vi "HP 3457A Address constant.vi"() -> ()   [LabVIEW 2020]
panel:
  in  "HP 3457A Address":string="22"
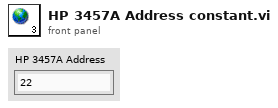
[diagram p1: front panel]
diagram:
